vi "_Raise Source Changed Event.vi"(4 "Display State In":T1, 5 "Event Data":cluster{"sender":refnum<k24>, "e":refnum<k24>}, 6 "Control Ref":refnum<k24>, 7 "Event Common Data":T2) -> ()   [LabVIEW 2020, in "WebView2 Control.xctl"]
uses:
  WebView2 Control.xctl
  E:/Labview/LV 2020/Libs/WebView2/LV-WebView2/Source/Libs/Microsoft.Web.WebView2.Core.dll
  Libs/Microsoft.Web.WebView2.Core.dll
  Events.ctl
  Navigation Event Data.ctl
  Source Changed Event Data.ctl
  Navigation Start Event Data.ctl
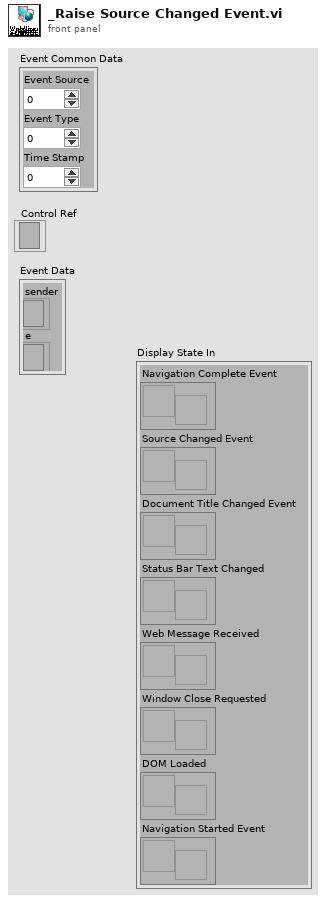
[diagram p1: front panel]
types:
  T1 = typedef "WebView2 Control.xctl/Events.ctl" = cluster{"Navigation Complete Event":refnum<user-event>, "Source Changed Event":refnum<user-event>, "Document Title Changed Event":refnum<user-event>, "Status Bar Text Changed":refnum<user-event>, "Web Message Received":refnum<user-event>, "Window Close Requested":refnum<user-event>, "DOM Loaded":refnum<user-event>, "Navigation Started Event":refnum<user-event>}
  T2 = cluster{"Event Source":i32, "Event Type":u32, "Time Stamp":u32}
  T3 = typedef "WebView2 Control.xctl/Source Changed Event Data.ctl" = cluster{"Source":string, "IsNewDocument":bool}
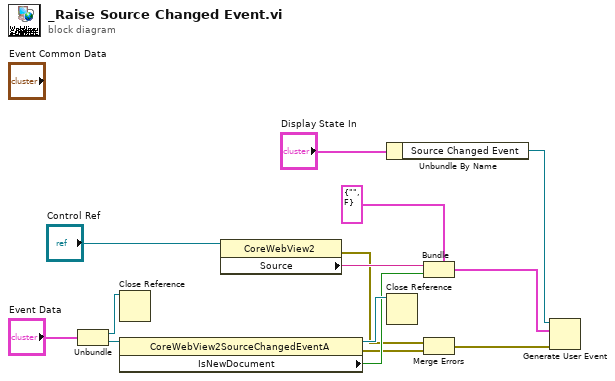
[diagram p0: block diagram]
diagram:
  n1 = Unbundle("Event Data") -> ("sender"=w10:refnum<k24>, "e"=w11:refnum<k24>)
  n2 = Close Reference(reference=w10) -> ()  [unwired: 1 in, 1 out]
  n3 = property class="CoreWebView2SourceChangedEventA"(reference=w11) -> (reference out=w8:refnum<k24>, error out=w3:errorcluster, "IsNewDocument"=w7:bool)  [unwired: 1 in]
  n4 = property class="CoreWebView2"(reference="Control Ref") -> (error out=w1:errorcluster, "Source"=w5:string)  [unwired: 1 in, 1 out]
  n5 = Unbundle By Name("Display State In") -> ("Source Changed Event"=w13:refnum<user-event>)
  n6 = Close Reference(reference=w8) -> ()  [unwired: 1 in, 1 out]
  n7 = Bundle(cluster=T3 {"Source"="", "IsNewDocument"=FALSE} ("output cluster"), "Source"=w5, "IsNewDocument"=w7) -> (w4:T3)
  n8 = Merge Errors(w1, w3) -> (w2:errorcluster)
  n9 = Generate User Event(user event=w13, event data cluster=w4, error in=w2) -> ()  [unwired: 1 in, 2 out]
